vi "Translator.File.SetFont.vi"(8 "error in":errorcluster, 11 "Translation file":path=path "c:/ni-rt.ini") -> (0 "error out":errorcluster, 2 "font name":string="abcdefghijklmnopqrstuvwxyz")   [LabVIEW 2010]
uses:
  <vilib>/Utility/config.llb/Read Key (String).vi
  <vilib>/Utility/config.llb/Write Key (String).vi
  <vilib>/Utility/config.llb/NI_LVConfig.lvlib
panel:
  out "Tahoma":string="abcdefghijklmnopqrstuvwxyz"
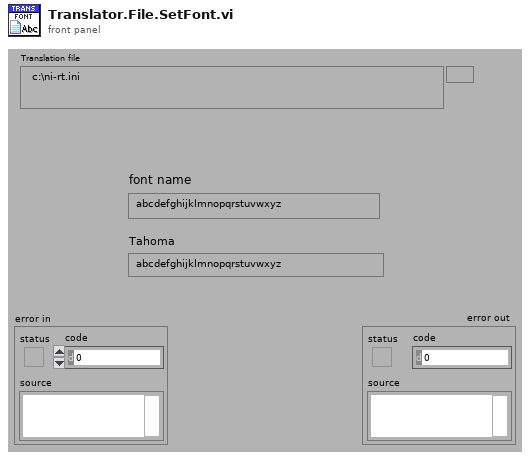
[diagram p1: front panel]
types:
  T1 = typedef "NI_LVConfig.lvlib/Config Data RefNum.ctl" = refnum<k1>
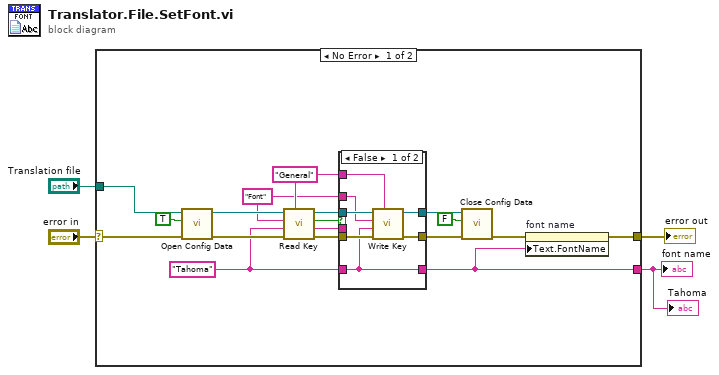
[diagram p0: block diagram]
diagram:
  n1 = case shown="No Error" "error in" {
    selector: "error in" -> [w15 w33]
    tunnel: [w16 w33] -> w4
    tunnel: "Translation file" -> [w18 _]
    tunnel: [w5 _] -> w1
    frame No Error {
      w6 = "Tahoma" ("default value")
      w8 = "Font" ("section")
      w9 = "General" ("section")
      n2 = call <vilib>:"Open Config Data.vi"("error in (no error)"=w15, "create file if necessary (T)"=TRUE, "configuration file path"=w18) -> ("error out"=w21:errorcluster, "refnum"=w20:T1)  [unwired: 6 in, 1 out]
      n3 = call-poly <vilib>:"Read Key.vi"("section"=w9, "error in (no error)"=w21, "default value"=w6, "key"=w8, "refnum"=w20) -> ("error out"=w13:errorcluster, "value"=w7:string, "found?"=w14:bool, "refnum out"=w10:T1)  [unwired: 3 in]
      n4 = case shown="False" w14 {
        tunnel: w13 -> [w29 w32]
        tunnel: [w28 w32] -> w12
        tunnel: [w27 w31] -> w11
        tunnel: w10 -> [w26 w31]
        tunnel: w9 -> [w25 _]
        tunnel: w8 -> [w24 _]
        tunnel: w7 -> [_ w30]
        tunnel: w6 -> [w23 _]
        tunnel: [w23 w30] -> w5
        frame False {
          n5 = call-poly <vilib>:"Write Key.vi"("section"=w25, "error in (no error)"=w29, "value"=w23, "key"=w24, "refnum"=w26) -> ("error out"=w28:errorcluster, "refnum out"=w27:T1)  [unwired: 4 in, 1 out]
        }
        frame True {
        }
      }
      n6 = call <vilib>:"Close Config Data.vi"("error in (no error)"=w12, "write file if changed (T)"=FALSE, "refnum"=w11) -> ("error out"=w17:errorcluster)  [unwired: 7 in, 1 out]
      n7 = property on="font name" class="Str"(error in=w17, "Text.FontName"=w5) -> (error out=w16:errorcluster)  [unwired: 1 in, 1 out]
    }
    frame Error {
    }
  }
  "error out" <- w4
  "font name" <- w1
  "Tahoma" <- w1
